vi "IIR Cascade DC Gain.vi"(4 "IIR Filter Cluster":T1={"filter structure"=enum."IIR 2nd Order", "Reverse Coefficients"=[0.0, 0.0], "Forward Coefficients"=[1.0, 0.0, 0.0]}) -> (1 "Gain":dbl)   [LabVIEW 2010]
panel:
  # "Find DC gain of an IIR cascade filter"
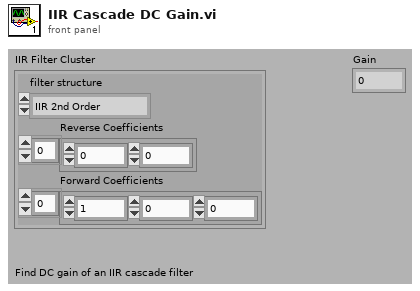
[diagram p1: front panel]
types:
  T1 = cluster{"filter structure":enum32{"IIR 2nd Order", "IIR 4th Order"}, "Reverse Coefficients":dbl[], "Forward Coefficients":dbl[]}
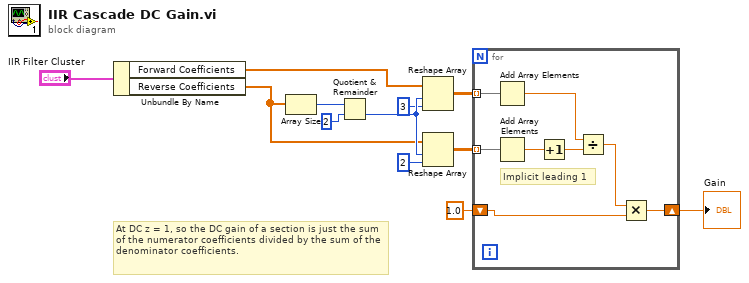
[diagram p0: block diagram]
diagram:
  # "At DC z = 1, so the DC gain of a section is just the sum of the numerator coefficients divided by the sum of the denominator coefficients."
  n1 = Unbundle By Name("IIR Filter Cluster") -> ("Forward Coefficients"=w2:dbl[], "Reverse Coefficients"=w1:dbl[])
  n2 = Array Size(array=w1) -> (size(s)=w10:i32)
  n3 = Quotient & Remainder(x=w10, y=2) -> (floor(x/y)=w11:i32)  [unwired: 1 out]
  n4 = Reshape Array(w2, w11, 3 ("dimension size")) -> (w6:dbl[][])
  n5 = Reshape Array(w1, w11, 2 ("dimension size")) -> (w5:dbl[][])
  n6 = for {
    tunnel: w6 -> [w19] mode=indexing
    tunnel: w5 -> [w18] mode=indexing
    shift-right: [w17] -> w3
    shift-left: 1.0 -> [w13]
    # "Implicit leading 1"
    n7 = Add Array Elements(numeric array=w19) -> (sum=w15:dbl)
    n8 = Add Array Elements(numeric array=w18) -> (sum=w20:dbl)
    n9 = Increment(x=w20) -> (x+1=w16:dbl)
    n10 = Divide(x=w15, y=w16) -> (x/y=w14:dbl)
    n11 = Multiply(x=w14, y=w13) -> (x*y=w17:dbl)
  }
  "Gain" <- w3
